vi "RemoteScopeSession_CallInitializeMeasurementLinkSessionWithAttachBehavior_RemoteSessionAttached.vi"(8 "error in":errorcluster) -> (0 "error out":errorcluster, 2 "result":string, 3 "pass":bool)   [LabVIEW 2020, in "MeasurementServerTests.lvlib"]
uses:
  MeasurementServerTests.lvlib
  Runtime/MeasurementLink Instrument/IInstrument/Initialize Session Behavior.ctl
  Runtime/MeasurementLink Instrument/IInstrument/IInstrument.lvclass
  Runtime/MeasurementLink niScope/Instrument/Instrument.lvclass
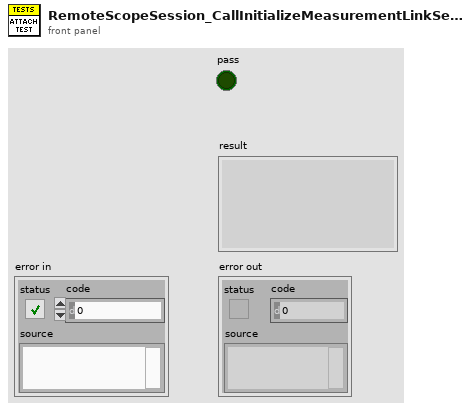
[diagram p1: front panel]
types:
  T1 = typedef "MeasurementLink Instrument.lvlib/IInstrument.lvclass/Remote Connection Options.ctl" = cluster{"session name":string, "address":string, "port":u32}
  T2 = typedef "MeasurementLink Instrument.lvlib/IInstrument.lvclass/Initialize Session Behavior.ctl" = enum16{"Create Session", "Attach Session"}
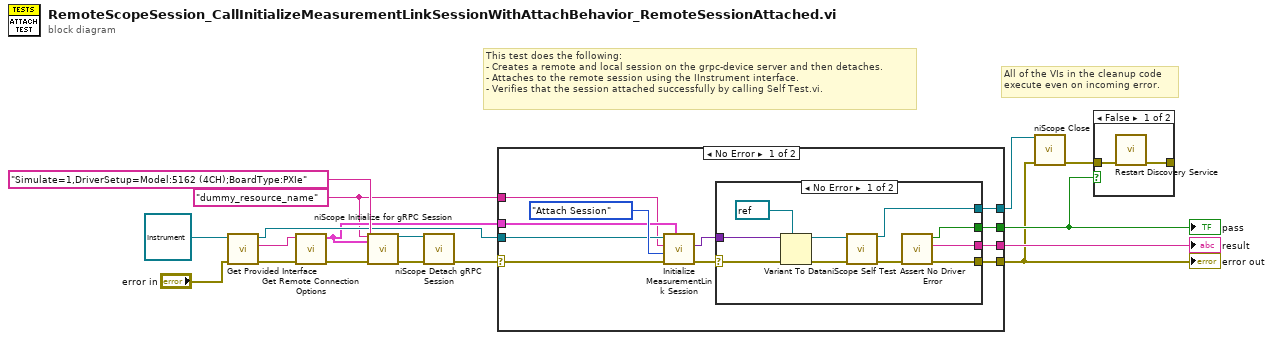
[diagram p0: block diagram]
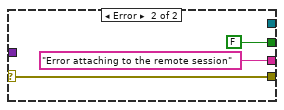
[diagram p2: hidden frame]
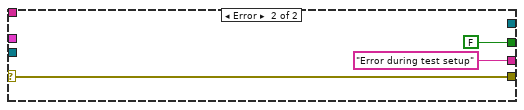
[diagram p3: hidden frame]
diagram:
  w1 = "dummy_resource_name" ("resource name")
  # "All of the VIs in the cleanup code\nexecute even on incoming error."
  # "This test does the following:\n- Creates a remote and local session on the grpc-device server and then detaches.\n- Attaches to the remote session using the IInstrument interface.\n- Verifies that the session attached successfully by calling Self Test.vi."
  n1 = call-dynamic "Get Provided Interface.vi"("error in"="error in", "instrument in"=refnum<class "Instrument.lvclass"> refnum ("MeasurementLink niScope.lvlib:Instrument.lvclass")) -> ("error out"=w9:errorcluster, "provided interface"=w8:string, "instrument out"=w6:refnum<class "Instrument.lvclass">)  [unwired: 7 in]
  n2 = call "Get Remote Connection Options.vi"("error in"=w9, "provided interface"=w8) -> ("error out"=w11:errorcluster, "remote connection options"=w2:T1)  [unwired: 8 in]
  n3 = call <instrlib>:"niScope Initialize for gRPC Session.vi"("resource name"=w1, "gRPC options"=w2, "option string"="Simulate=1,DriverSetup=Model:5162 (4CH);BoardType:PXIe", "error in"=w11) -> ("instrument handle"=w3:refnum<k15>, "error out"=w5:errorcluster)  [unwired: 10 in]
  n4 = call <instrlib>:"niScope Detach gRPC Session.vi"("instrument handle"=w3, "error in"=w5) -> ("error out"=w4:errorcluster)  [unwired: 13 in]
  n5 = case shown="No Error" w4 {
    selector: w4 -> [w22 w42]
    tunnel: [w27 w42] -> w13
    tunnel: [w28 FALSE] -> w14
    tunnel: [w26 "Error during test setup" ("f")] -> w17
    tunnel: w6 -> [w21 _]
    tunnel: [w20 _] -> w16
    tunnel: w2 -> [w19 _]
    tunnel: w1 -> [w18 _]
    frame No Error {
      n6 = call-dynamic "Initialize MeasurementLink Session.vi"("remote connection options"=w19, "error in"=w22, "initialize session behavior"=Initialize_Session_Behavior."Attach Session", "resource name"=w18, "instrument in"=w21) -> ("error out"=w24:errorcluster, "session out"=w25:variant)  [unwired: 4 in, 1 out]
      n7 = case shown="No Error" w24 {
        selector: w24 -> [w37 w40]
        tunnel: [w33 FALSE] -> w28
        tunnel: [w31 w40] -> w27
        tunnel: [w32 "Error attaching to the remote session"] -> w26
        tunnel: w25 -> [w38 _]
        tunnel: [w35 _] -> w20
        frame No Error {
          n8 = Variant To Data(error in=w37, type=refnum<k15> refnum ("instrument handle"), Variant=w38) -> (data=w29:refnum<k15>, error out=w36:errorcluster)
          n9 = call <instrlib>:"niScope Self Test.vi"("instrument handle"=w29, "error in"=w36) -> ("instrument handle out"=w35:refnum<k15>, "error out"=w34:errorcluster)  [unwired: 10 in, 2 out]
          n10 = call "Assert No Driver Error.vi"("error in"=w34) -> ("error out"=w31:errorcluster, "result"=w32:string, "pass?"=w33:bool)  [unwired: 8 in]
        }
        frame Error {
        }
      }
    }
    frame Error {
    }
  }
  "error out" <- w13
  "pass" <- w14
  "result" <- w17
  n11 = call <instrlib>:"niScope Close.vi"("instrument handle"=w16, "error in"=w13) -> ("error out"=w15:errorcluster)  [unwired: 13 in]
  n12 = case shown="False" w14 {
    tunnel: w15 -> [w46 _]
    tunnel: [w45 _] -> _
    frame False {
      n13 = call "Restart Discovery Service.vi"("error in"=w46) -> ("error out"=w45:errorcluster)  [unwired: 10 in]
    }
    frame True {
    }
  }
